vi "Get dt.vi"(8 "error in (no error)":errorcluster, 11 "Waveform Receive in":refnum<class "Waveform Receive.lvclass">) -> (0 "error out":errorcluster, 1 "dt Changed?":bool, 2 "dt":dbl, 3 "Waveform Receive out":refnum<class "Waveform Receive.lvclass">)   [LabVIEW 2015, in "Waveform Data Logger Engine.lvlib" / "Waveform Receive.lvclass"]
uses:
  Waveform Receive.lvclass
  Waveform Receive.lvclass/Waveform Receive.ctl
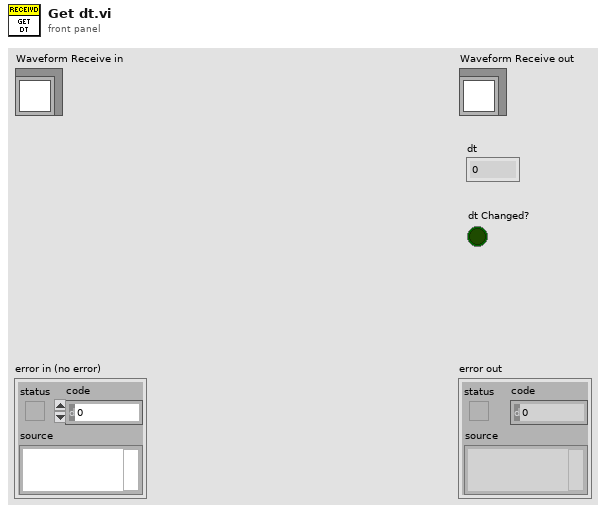
[diagram p1: front panel]
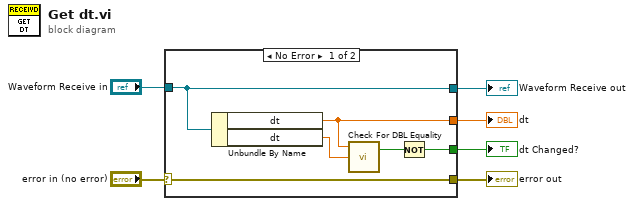
[diagram p0: block diagram]
diagram:
  n1 = case shown="No Error" "error in (no error)" {
    selector: "error in (no error)" -> [w12 w14]
    tunnel: [w12 w14] -> w5
    tunnel: [w11 w13] -> w3
    tunnel: "Waveform Receive in" -> [w11 w13]
    tunnel: [w10 _] -> w2
    tunnel: [w7 _] -> w1
    frame No Error {
      n2 = Unbundle By Name(w11) -> ("dt"=w10:dbl, "dt"=w9:dbl)
      n3 = call "Check For DBL Equality.vi"("n2"=w9, "n1"=w10) -> ("equal?"=w8:bool)  [unwired: 2 in]
      n4 = Not(x=w8) -> (.not. x?=w7:bool)
    }
    frame Error {
    }
  }
  "error out" <- w5
  "Waveform Receive out" <- w3
  "dt Changed?" <- w1
  "dt" <- w2
